vi "DIOs.vi"(0 "Mod6/DIOs":T1, 1 "Mod5/DIOs":T2) -> ()   [LabVIEW 2010]
uses:
  <vilib>/eio/EIONode/EIONode.xnode
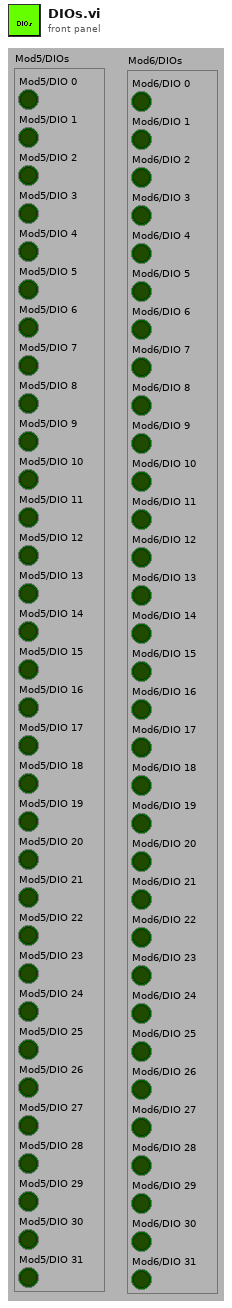
[diagram p1: front panel]
types:
  T1 = cluster{"Mod6/DIO 0":bool, "Mod6/DIO 1":bool, "Mod6/DIO 2":bool, "Mod6/DIO 3":bool, "Mod6/DIO 4":bool, "Mod6/DIO 5":bool, "Mod6/DIO 6":bool, "Mod6/DIO 7":bool, "Mod6/DIO 8":bool, "Mod6/DIO 9":bool, "Mod6/DIO 10":bool, "Mod6/DIO 11":bool, "Mod6/DIO 12":bool, "Mod6/DIO 13":bool, "Mod6/DIO 14":bool, "Mod6/DIO 15":bool, "Mod6/DIO 16":bool, "Mod6/DIO 17":bool, "Mod6/DIO 18":bool, "Mod6/DIO 19":bool, "Mod6/DIO 20":bool, "Mod6/DIO 21":bool, "Mod6/DIO 22":bool, "Mod6/DIO 23":bool, "Mod6/DIO 24":bool, "Mod6/DIO 25":bool, "Mod6/DIO 26":bool, "Mod6/DIO 27":bool, "Mod6/DIO 28":bool, "Mod6/DIO 29":bool, "Mod6/DIO 30":bool, "Mod6/DIO 31":bool}
  T2 = cluster{"Mod5/DIO 0":bool, "Mod5/DIO 1":bool, "Mod5/DIO 2":bool, "Mod5/DIO 3":bool, "Mod5/DIO 4":bool, "Mod5/DIO 5":bool, "Mod5/DIO 6":bool, "Mod5/DIO 7":bool, "Mod5/DIO 8":bool, "Mod5/DIO 9":bool, "Mod5/DIO 10":bool, "Mod5/DIO 11":bool, "Mod5/DIO 12":bool, "Mod5/DIO 13":bool, "Mod5/DIO 14":bool, "Mod5/DIO 15":bool, "Mod5/DIO 16":bool, "Mod5/DIO 17":bool, "Mod5/DIO 18":bool, "Mod5/DIO 19":bool, "Mod5/DIO 20":bool, "Mod5/DIO 21":bool, "Mod5/DIO 22":bool, "Mod5/DIO 23":bool, "Mod5/DIO 24":bool, "Mod5/DIO 25":bool, "Mod5/DIO 26":bool, "Mod5/DIO 27":bool, "Mod5/DIO 28":bool, "Mod5/DIO 29":bool, "Mod5/DIO 30":bool, "Mod5/DIO 31":bool}
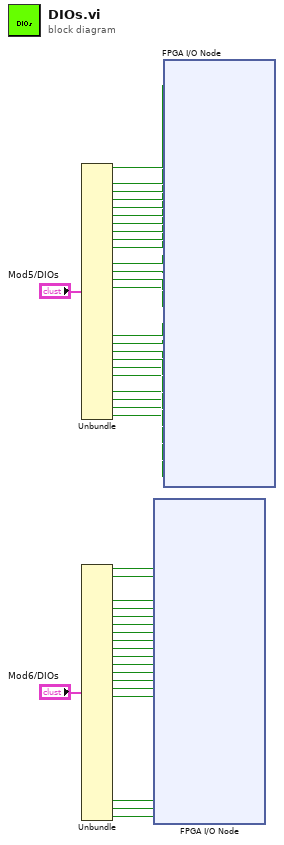
[diagram p0: block diagram]
diagram:
  n1 = Unbundle("Mod5/DIOs") -> ("Mod5/DIO 0"=w43:bool, "Mod5/DIO 2"=w42:bool, "Mod5/DIO 3"=w41:bool, "Mod5/DIO 4"=w40:bool, "Mod5/DIO 5"=w39:bool, "Mod5/DIO 6"=w38:bool, "Mod5/DIO 7"=w37:bool, "Mod5/DIO 8"=w36:bool, "Mod5/DIO 9"=w35:bool, "Mod5/DIO 10"=w34:bool, "Mod5/DIO 12"=w33:bool, "Mod5/DIO 13"=w32:bool, "Mod5/DIO 14"=w31:bool, "Mod5/DIO 15"=w30:bool, "Mod5/DIO 21"=w29:bool, "Mod5/DIO 22"=w28:bool, "Mod5/DIO 23"=w27:bool, "Mod5/DIO 24"=w26:bool, "Mod5/DIO 25"=w25:bool, "Mod5/DIO 26"=w24:bool, "Mod5/DIO 28"=w23:bool, "Mod5/DIO 29"=w22:bool, "Mod5/DIO 30"=w21:bool, "Mod5/DIO 31"=w20:bool)  [unwired: 8 out]
  n2 = Unbundle("Mod6/DIOs") -> ("Mod6/DIO 0"=w18:bool, "Mod6/DIO 1"=w17:bool, "Mod6/DIO 4"=w16:bool, "Mod6/DIO 5"=w15:bool, "Mod6/DIO 6"=w14:bool, "Mod6/DIO 7"=w13:bool, "Mod6/DIO 8"=w12:bool, "Mod6/DIO 9"=w11:bool, "Mod6/DIO 10"=w10:bool, "Mod6/DIO 11"=w9:bool, "Mod6/DIO 12"=w8:bool, "Mod6/DIO 13"=w7:bool, "Mod6/DIO 14"=w6:bool, "Mod6/DIO 15"=w5:bool, "Mod6/DIO 16"=w4:bool, "Mod6/DIO 29"=w3:bool, "Mod6/DIO 30"=w2:bool, "Mod6/DIO 31"=w1:bool)  [unwired: 14 out]
  n3 = xnode "FPGA I/O Node"("Mod6/DIO0"=w18, "Mod6/DIO1"=w17, "Mod6/DIO4"=w16, "Mod6/DIO5"=w15, "Mod6/DIO6"=w14, "Mod6/DIO7"=w13, "Mod6/DIO8"=w12, "Mod6/DIO9"=w11, "Mod6/DIO10"=w10, "Mod6/DIO11"=w9, "Mod6/DIO12"=w8, "Mod6/DIO13"=w7, "Mod6/DIO14"=w6, "Mod6/DIO15"=w5, "Mod6/DIO16"=w4, "Mod6/DIO29"=w3, "Mod6/DIO30"=w2, "Mod6/DIO31"=w1) -> ()  [unwired: 18 in, 18 out]
  n4 = xnode "FPGA I/O Node"("Mod5/DIO0"=w43, "Mod5/DIO2"=w42, "Mod5/DIO3"=w41, "Mod5/DIO4"=w40, "Mod5/DIO5"=w39, "Mod5/DIO6"=w38, "Mod5/DIO7"=w37, "Mod5/DIO8"=w36, "Mod5/DIO9"=w35, "Mod5/DIO10"=w34, "Mod5/DIO12"=w33, "Mod5/DIO13"=w32, "Mod5/DIO14"=w31, "Mod5/DIO15"=w30, "Mod5/DIO21"=w29, "Mod5/DIO22"=w28, "Mod5/DIO23"=w27, "Mod5/DIO24"=w26, "Mod5/DIO25"=w25, "Mod5/DIO26"=w24, "Mod5/DIO28"=w23, "Mod5/DIO29"=w22, "Mod5/DIO30"=w21, "Mod5/DIO31"=w20) -> ()  [unwired: 24 in, 24 out]
